vi "Row Pattern.vi"(8 "error in (no error)":errorcluster, 11 "Grid Animation in":refnum<class "Grid Animation.lvclass">) -> (0 "error out":errorcluster, 3 "Grid Animation out":refnum<class "Grid Animation.lvclass">)   [LabVIEW 2021, in "Grid Animation.lvlib" / "Grid Animation.lvclass"]
uses:
  Grid Animation.lvclass
  Grid Animation.lvclass/Grid Animation.ctl
  <vilib>/ActorFramework/Message Enqueuer/Init from Existing Queue.vi
  <vilib>/ActorFramework/Message Enqueuer/Message Enqueuer.lvclass
  <vilib>/ActorFramework/Actor/Actor.lvclass
  C:/Program Files/National Instruments/LabVIEW 2024/vi.lib/ActorFramework/Actor/Actor.lvclass
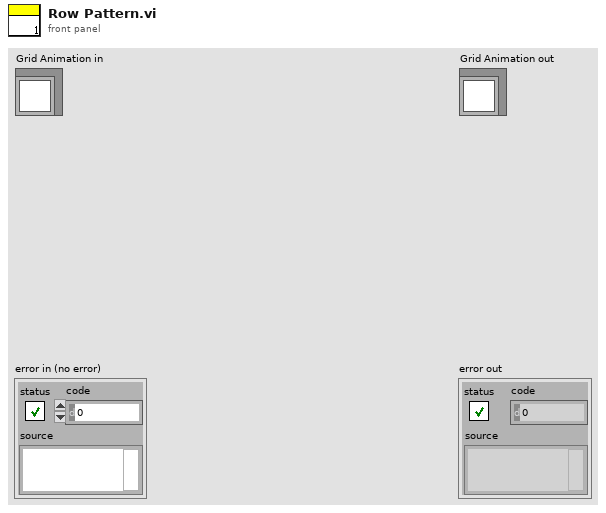
[diagram p1: front panel]
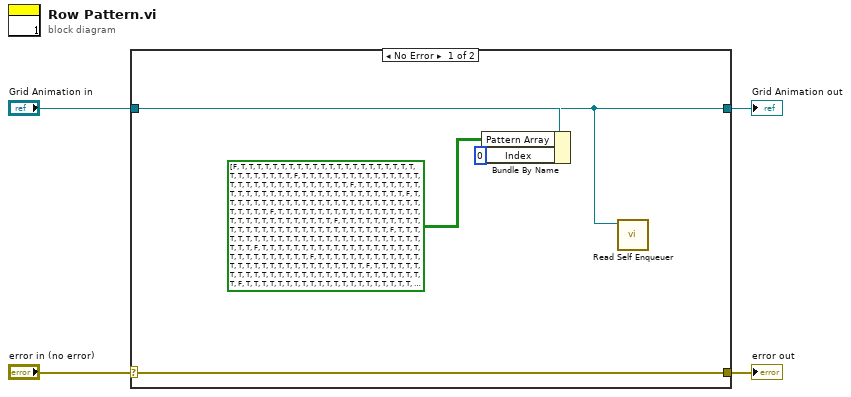
[diagram p0: block diagram]
diagram:
  n1 = case shown="No Error" "error in (no error)" {
    selector: "error in (no error)" -> [w9 w11]
    tunnel: [w9 w11] -> w3
    tunnel: [w5 w10] -> w1
    tunnel: "Grid Animation in" -> [w8 w10]
    frame No Error {
      n2 = Bundle By Name(cluster=w8, "Pattern Array"=bool[][][] [[[FALSE, TRUE, TRUE, TRUE, TRUE, TRUE], [TRUE, TRUE, TRUE, TRUE, TRUE, TRUE], [TRUE, TRUE, TRUE, TRUE, TRUE, TRUE], [TRUE, TRUE, TRUE, TRUE, TRUE, TRUE], [TRUE, TRUE, TRUE, TRUE, TRUE, TRUE]], [[TRUE, FALSE, TRUE, TRUE, TRUE, TRUE], [TRUE, TRUE, TRUE, TRUE, TRUE, TRUE], [TRUE, TRUE, TRUE, TRUE, TRUE, TRUE], [TRUE, TRUE, TRUE, TRUE, TRUE, TRUE], [TRUE, TRUE, TRUE, TRUE, TRUE, TRUE]], [[TRUE, TRUE, FALSE, TRUE, TRUE, TRUE], [TRUE, TRUE, TRUE, TRUE, TRUE, TRUE], [TRUE, TRUE, TRUE, TRUE, TRUE, TRUE], [TRUE, TRUE, TRUE, TRUE, TRUE, TRUE], [TRUE, TRUE, TRUE, TRUE, TRUE, TRUE]], [[TRUE, TRUE, TRUE, FALSE, TRUE, TRUE], [TRUE, TRUE, TRUE, TRUE, TRUE, TRUE], [TRUE, TRUE, TRUE, TRUE, TRUE, TRUE], [TRUE, TRUE, TRUE, TRUE, TRUE, TRUE], [TRUE, TRUE, TRUE, TRUE, TRUE, TRUE]], [[TRUE, TRUE, TRUE, TRUE, FALSE, TRUE], [TRUE, TRUE, TRUE, TRUE, TRUE, TRUE], [TRUE, TRUE, TRUE, TRUE, TRUE, TRUE], [TRUE, TRUE, TRUE, TRUE, TRUE, TRUE], [TRUE, TRUE, TRUE, TRUE, TRUE, TRUE]], [[TRUE, TRUE, TRUE, TRUE, TRUE, TRUE], [FALSE, TRUE, TRUE, TRUE, TRUE, TRUE], [TRUE, TRUE, TRUE, TRUE, TRUE, TRUE], [TRUE, TRUE, TRUE, TRUE, TRUE, TRUE], [TRUE, TRUE, TRUE, TRUE, TRUE, TRUE]], [[TRUE, TRUE, TRUE, TRUE, TRUE, TRUE], [TRUE, FALSE, TRUE, TRUE, TRUE, TRUE], [TRUE, TRUE, TRUE, TRUE, TRUE, TRUE], [TRUE, TRUE, TRUE, TRUE, TRUE, TRUE], [TRUE, TRUE, TRUE, TRUE, TRUE, TRUE]], [[TRUE, TRUE, TRUE, TRUE, TRUE, TRUE], [TRUE, TRUE, FALSE, TRUE, TRUE, TRUE], [TRUE, TRUE, TRUE, TRUE, TRUE, TRUE], [TRUE, TRUE, TRUE, TRUE, TRUE, TRUE], [TRUE, TRUE, TRUE, TRUE, TRUE, TRUE]], [[TRUE, TRUE, TRUE, TRUE, TRUE, TRUE], [TRUE, TRUE, TRUE, FALSE, TRUE, TRUE], [TRUE, TRUE, TRUE, TRUE, TRUE, TRUE], [TRUE, TRUE, TRUE, TRUE, TRUE, TRUE], [TRUE, TRUE, TRUE, TRUE, TRUE, TRUE]], [[TRUE, TRUE, TRUE, TRUE, TRUE, TRUE], [TRUE, TRUE, TRUE, TRUE, FALSE, TRUE], [TRUE, TRUE, TRUE, TRUE, TRUE, TRUE], [TRUE, TRUE, TRUE, TRUE, TRUE, TRUE], [TRUE, TRUE, TRUE, TRUE, TRUE, TRUE]], [[TRUE, TRUE, TRUE, TRUE, TRUE, TRUE], [TRUE, TRUE, TRUE, TRUE, TRUE, TRUE], [FALSE, TRUE, TRUE, TRUE, TRUE, TRUE], [TRUE, TRUE, TRUE, TRUE, TRUE, TRUE], [TRUE, TRUE, TRUE, TRUE, TRUE, TRUE]], [[TRUE, TRUE, TRUE, TRUE, TRUE, TRUE], [TRUE, TRUE, TRUE, TRUE, TRUE, TRUE], [TRUE, FALSE, TRUE, TRUE, TRUE, TRUE], [TRUE, TRUE, TRUE, TRUE, TRUE, TRUE], [TRUE, TRUE, TRUE, TRUE, TRUE, TRUE]], [[TRUE, TRUE, TRUE, TRUE, TRUE, TRUE], [TRUE, TRUE, TRUE, TRUE, TRUE, TRUE], [TRUE, TRUE, FALSE, TRUE, TRUE, TRUE], [TRUE, TRUE, TRUE, TRUE, TRUE, TRUE], [TRUE, TRUE, TRUE, TRUE, TRUE, TRUE]], [[TRUE, TRUE, TRUE, TRUE, TRUE, TRUE], [TRUE, TRUE, TRUE, TRUE, TRUE, TRUE], [TRUE, TRUE, TRUE, FALSE, TRUE, TRUE], [TRUE, TRUE, TRUE, TRUE, TRUE, TRUE], [TRUE, TRUE, TRUE, TRUE, TRUE, TRUE]], [[TRUE, TRUE, TRUE, TRUE, TRUE, TRUE], [TRUE, TRUE, TRUE, TRUE, TRUE, TRUE], [TRUE, TRUE, TRUE, TRUE, FALSE, TRUE], [TRUE, TRUE, TRUE, TRUE, TRUE, TRUE], [TRUE, TRUE, TRUE, TRUE, TRUE, TRUE]], [[TRUE, TRUE, TRUE, TRUE, TRUE, TRUE], [TRUE, TRUE, TRUE, TRUE, TRUE, TRUE], [TRUE, TRUE, TRUE, TRUE, TRUE, TRUE], [FALSE, TRUE, TRUE, TRUE, TRUE, TRUE], [TRUE, TRUE, TRUE, TRUE, TRUE, TRUE]], [[TRUE, TRUE, TRUE, TRUE, TRUE, TRUE], [TRUE, TRUE, TRUE, TRUE, TRUE, TRUE], [TRUE, TRUE, TRUE, TRUE, TRUE, TRUE], [TRUE, FALSE, TRUE, TRUE, TRUE, TRUE], [TRUE, TRUE, TRUE, TRUE, TRUE, TRUE]], [[TRUE, TRUE, TRUE, TRUE, TRUE, TRUE], [TRUE, TRUE, TRUE, TRUE, TRUE, TRUE], [TRUE, TRUE, TRUE, TRUE, TRUE, TRUE], [TRUE, TRUE, FALSE, TRUE, TRUE, TRUE], [TRUE, TRUE, TRUE, TRUE, TRUE, TRUE]], [[TRUE, TRUE, TRUE, TRUE, TRUE, TRUE], [TRUE, TRUE, TRUE, TRUE, TRUE, TRUE], [TRUE, TRUE, TRUE, TRUE, TRUE, TRUE], [TRUE, TRUE, TRUE, FALSE, TRUE, TRUE], [TRUE, TRUE, TRUE, TRUE, TRUE, TRUE]], [[TRUE, TRUE, TRUE, TRUE, TRUE, TRUE], [TRUE, TRUE, TRUE, TRUE, TRUE, TRUE], [TRUE, TRUE, TRUE, TRUE, TRUE, TRUE], [TRUE, TRUE, TRUE, TRUE, FALSE, TRUE], [TRUE, TRUE, TRUE, TRUE, TRUE, TRUE]], [[TRUE, TRUE, TRUE, TRUE, TRUE, TRUE], [TRUE, TRUE, TRUE, TRUE, TRUE, TRUE], [TRUE, TRUE, TRUE, TRUE, TRUE, TRUE], [TRUE, TRUE, TRUE, TRUE, TRUE, TRUE], [FALSE, TRUE, TRUE, TRUE, TRUE, TRUE]], [[TRUE, TRUE, TRUE, TRUE, TRUE, TRUE], [TRUE, TRUE, TRUE, TRUE, TRUE, TRUE], [TRUE, TRUE, TRUE, TRUE, TRUE, TRUE], [TRUE, TRUE, TRUE, TRUE, TRUE, TRUE], [TRUE, FALSE, TRUE, TRUE, TRUE, TRUE]], [[TRUE, TRUE, TRUE, TRUE, TRUE, TRUE], [TRUE, TRUE, TRUE, TRUE, TRUE, TRUE], [TRUE, TRUE, TRUE, TRUE, TRUE, TRUE], [TRUE, TRUE, TRUE, TRUE, TRUE, TRUE], [TRUE, TRUE, FALSE, TRUE, TRUE, TRUE]], [[TRUE, TRUE, TRUE, TRUE, TRUE, TRUE], [TRUE, TRUE, TRUE, TRUE, TRUE, TRUE], [TRUE, TRUE, TRUE, TRUE, TRUE, TRUE], [TRUE, TRUE, TRUE, TRUE, TRUE, TRUE], [TRUE, TRUE, TRUE, FALSE, TRUE, TRUE]], [[TRUE, TRUE, TRUE, TRUE, TRUE, TRUE], [TRUE, TRUE, TRUE, TRUE, TRUE, TRUE], [TRUE, TRUE, TRUE, TRUE, TRUE, TRUE], [TRUE, TRUE, TRUE, TRUE, TRUE, TRUE], [TRUE, TRUE, TRUE, TRUE, FALSE, TRUE]]], "Index"=0) -> (w5:refnum<class "Grid Animation.lvclass">)
      n3 = call <vilib>:"Read Self Enqueuer.vi"("Actor"=w5) -> ()  [unwired: 10 in, 1 out]
    }
    frame Error {
    }
  }
  "error out" <- w3
  "Grid Animation out" <- w1
